vi "DAQ_Init.vi"(8 "error in":errorcluster caption="entrée d'erreur", 9 "RegenMode":i32(ring)=10097 items=["Allow Regeneration"=10097, "Do Not Allow Regeneration"=10158], 10 "samples per channel":i32=1000, 11 "sample mode":i32(ring)=10123 items=["Échantillons finis"=10178, "Échantillons continus"=10123, "Point par point avec cadencement matériel"=12522]) -> (0 "error out":errorcluster caption="sortie d'erreur")   [LabVIEW 2025]
uses:
  <vilib>/DAQmx/create/channels.llb/DAQmx Create Channel (CO-Pulse Generation-Frequency).vi
  <vilib>/DAQmx/create/channels.llb/DAQmx Create Channel (DO-Digital Output).vi
  <vilib>/DAQmx/create/channels.llb/DAQmx Create Channel (AO-Voltage-Basic).vi
  <resource>/objmgr/daqmx.rc
  Controls/TypeDef_FGV.ctl
  <vilib>/DAQmx/configure/timing.llb/DAQmx Timing (Implicit).vi
  <vilib>/DAQmx/configure/timing.llb/DAQmx Timing (Sample Clock).vi
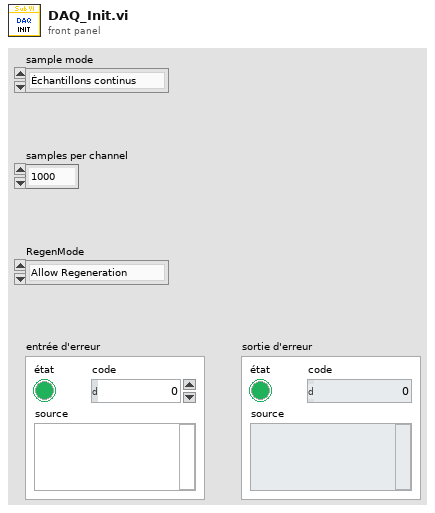
[diagram p1: front panel]
types:
  T1 = typedef "TypeDef_FGV.ctl" = enum16{"Initialize", "Write", "Read"}
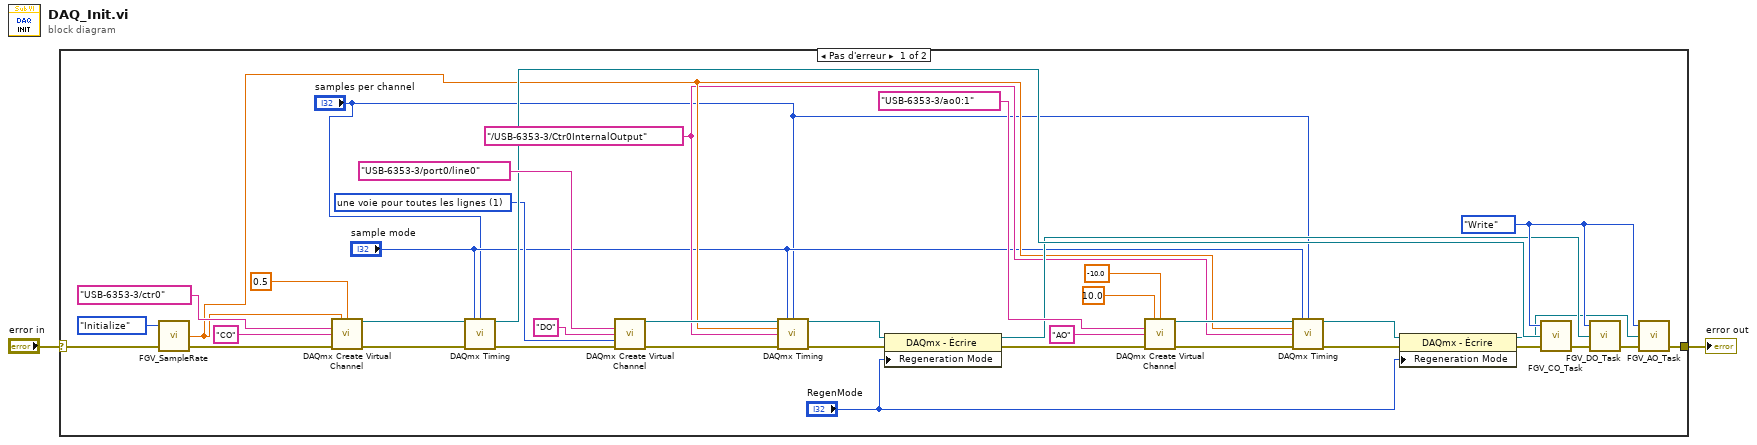
[diagram p0: block diagram]
diagram:
  n1 = case shown="Pas d'erreur" "error in" {
    selector: "error in" -> [w24 w41]
    tunnel: [w27 w41] -> w1
    frame No Error {
      w20 = 1 items=["une voie par ligne", "une voie pour toutes les lignes"] ("line grouping")
      w26 = TypeDef_FGV."Write" ("Action")
      w9 = tag "/USB-6353-3/Ctr0InternalOutput" ("HorlÉchant.Src")
      n2 = call "FGV_SampleRate.vi"("error in"=w24, "Action"=TypeDef_FGV."Initialize") -> ("error out"=w23:errorcluster, "CO task"=w10:dbl)  [unwired: 2 in]
      n3 = call-poly <vilib>:"DAQmx Create Virtual Channel.vi"("frequency"=w10, "duty cycle"=0.5, "counter"=tag "USB-6353-3/ctr0", "name to assign"="CO", "error in"=w23) -> ("task out"=w37:refnum<k21>, "error out"=w38:errorcluster)  [unwired: 9 in]
      n4 = call-poly <vilib>:"DAQmx Timing.vi"("task/channels in"=w37, "sample mode"="sample mode", "samples per channel"="samples per channel", "error in"=w38) -> ("task out"=w25:refnum<k21>, "error out"=w21:errorcluster)  [unwired: 10 in]
      n5 = call-poly <vilib>:"DAQmx Create Virtual Channel.vi"("lines"=tag "USB-6353-3/port0/line0", "name to assign"="DO", "line grouping"=w20, "error in"=w21) -> ("task out"=w17:refnum<k21>, "error out"=w16:errorcluster)  [unwired: 10 in]
      n6 = call-poly <vilib>:"DAQmx Timing.vi"("task/channels in"=w17, "sample mode"="sample mode", "samples per channel"="samples per channel", "rate"=w10, "source"=w9, "error in"=w16) -> ("task out"=w14:refnum<k21>, "error out"=w15:errorcluster)  [unwired: 8 in]
      n7 = property class="DAQmx - Écrire"(reference=w14, error in=w15, "Regeneration Mode"="RegenMode") -> (reference out=w19:refnum<k21>, error out=w18:errorcluster)
      n8 = call-poly <vilib>:"DAQmx Create Virtual Channel.vi"("maximum value"=10.0, "minimum value"=-10.0, "physical channels"=tag "USB-6353-3/ao0:1", "name to assign"="AO", "error in"=w18) -> ("task out"=w12:refnum<k21>, "error out"=w11:errorcluster)  [unwired: 9 in]
      n9 = call-poly <vilib>:"DAQmx Timing.vi"("task/channels in"=w12, "sample mode"="sample mode", "samples per channel"="samples per channel", "rate"=w10, "source"=w9, "error in"=w11) -> ("task out"=w8:refnum<k21>, "error out"=w13:errorcluster)  [unwired: 8 in]
      n10 = property class="DAQmx - Écrire"(reference=w8, error in=w13, "Regeneration Mode"="RegenMode") -> (reference out=w5:refnum<k21>, error out=w6:errorcluster)
      n11 = call "FGV_CO_Task.vi"("error in"=w6, "task out 2"=w25, "Action"=w26) -> ("error out"=w29:errorcluster)  [unwired: 1 in, 1 out]
      n12 = call "FGV_DO_Task.vi"("error in"=w29, "task out 2"=w19, "Action"=w26) -> ("error out"=w28:errorcluster)  [unwired: 1 in, 1 out]
      n13 = call "FGV_AO_Task.vi"("error in"=w28, "task out 2"=w5, "Action"=w26) -> ("error out"=w27:errorcluster)  [unwired: 1 in, 1 out]
    }
    frame Error {
    }
  }
  "error out" <- w1
